vi "Simple Adder Program.vi"() -> ()   [LabVIEW 2018]
uses:
  <vilib>/RTI DDS Toolkit/Types/RTI DDS Advanced Reader Configuration.ctl
  <vilib>/RTI DDS Toolkit/Types/RTI DDS Advanced Writer Configuration.ctl
  <vilib>/RTI DDS Toolkit/VIs/AdvancedCreateWriter_NumI32.vi
  <vilib>/RTI DDS Toolkit/VIs/Write_NumI32.vi
  <vilib>/RTI DDS Toolkit/VIs/AdvancedCreateReader_NumI32.vi
  <vilib>/RTI DDS Toolkit/VIs/Read_NumI32.vi
  <vilib>/RTI DDS Toolkit/Library/LVDDS_library.lvlib
panel:
  out "Int to ROS":i32=7
  in  "error in (no error) 2":errorcluster
  in  "Advanced Writer Configuration":T1={"typeName"="std_msgs::msg::dds_::Int32_", "keyName"="", "domainParticipantQoSProfile"="", "dataWriterQoSProfile"="", "forceArrayMapping?"=FALSE, "forceUnboundedString?"=FALSE}
  in  "stop":bool
  out "Int from ros":i32
  in  "error in (no error)":errorcluster
  in  "Advanced Reader Configuration":T2={"typeName"="std_msgs::msg::dds_::Int32_", "keyName"="", "domainParticipantQoSProfile"="", "dataReaderQoSProfile"="", "forceArrayMapping?"=FALSE, "forceExclusiveReader?"=FALSE, "forceRead? (only ExclusiveReader)"=FALSE, "forceUnboundedString?"=FALSE}
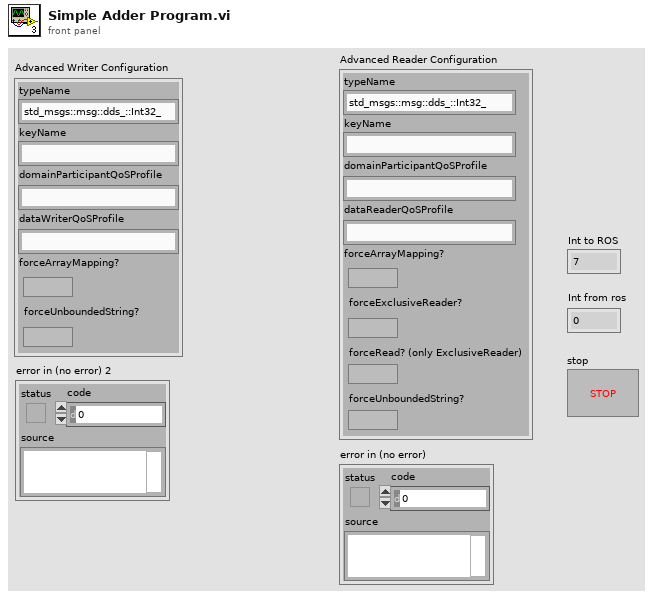
[diagram p1: front panel]
types:
  T1 = typedef "LVDDS_library.lvlib/RTI DDS Advanced Writer Configuration.ctl" = cluster{"typeName":string, "keyName":string, "domainParticipantQoSProfile":string, "dataWriterQoSProfile":string, "forceArrayMapping?":bool, "forceUnboundedString?":bool}
  T2 = typedef "LVDDS_library.lvlib/RTI DDS Advanced Reader Configuration.ctl" = cluster{"typeName":string, "keyName":string, "domainParticipantQoSProfile":string, "dataReaderQoSProfile":string, "forceArrayMapping?":bool, "forceExclusiveReader?":bool, "forceRead? (only ExclusiveReader)":bool, "forceUnboundedString?":bool}
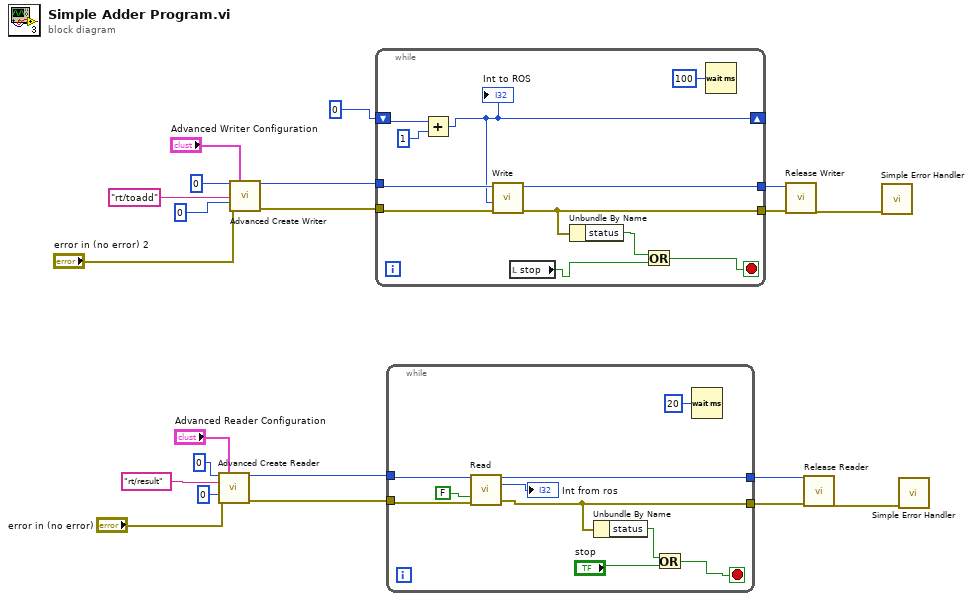
[diagram p0: block diagram]
diagram:
  n1 = call-poly <vilib>:"Advanced Create Reader.vi"("Domain Id"=u32 0 ("Domain id"), "Advanced Reader Configuration"="Advanced Reader Configuration", "Topic Name"="rt/result", "Data Type"=0, "error in (no error)"="error in (no error)") -> ("DDS Object Ref"=w16:u64, "error out"=w15:errorcluster)  [unwired: 9 in]
  n2 = call-poly <vilib>:"Advanced Create Writer.vi"("Domain Id"=u32 0, "Advanced Writer Configuration"="Advanced Writer Configuration", "Topic Name"="rt/toadd", "Data Type"=0, "error in (no error)"="error in (no error) 2") -> ("DDS Object Ref"=w5:u64, "error out"=w4:errorcluster)  [unwired: 9 in]
  n3 = while {
    shift-right: [w27] -> _
    shift-left: 0 -> [w31]
    tunnel: w5 -> [w29]
    tunnel: w4 -> [w28]
    tunnel: [w26] -> w3
    tunnel: [w25] -> w2
    stop <- w23 stop-if-true
    n4 = Add(x=w31, y=1) -> (x+y=w27:i32)
    "Int to ROS" <- w27
    n5 = call-poly <vilib>:"Write.vi"("error in (no error)"=w28, "Data"=w27, "DDS Object Ref in"=w29) -> ("error out"=w25:errorcluster, "DDS Object Ref out"=w26:u64)  [unwired: 7 in]
    n6 = local read "stop"() -> (w22:bool)
    n7 = Unbundle By Name "Unbundle By Name"(w25) -> ("status"=w24:bool)
    n8 = Or(x=w24, y=w22) -> (x .or. y?=w23:bool)
    n9 = Wait (ms)(milliseconds to wait=u32 100) -> ()  [unwired: 1 out]
  }
  n10 = while {
    tunnel: w16 -> [w42]
    tunnel: w15 -> [w41]
    tunnel: [w38] -> w14
    tunnel: [w37] -> w13
    stop <- w34 stop-if-true
    n11 = call-poly <vilib>:"Read.vi"("DDS Object Ref in"=w42, "Only New Samples"=FALSE, "error in (no error)"=w41) -> ("DDS Object Ref out"=w38:u64, "Data"=→"Int from ros":i32, "error out"=w37:errorcluster)  [unwired: 8 in, 2 out]
    n12 = Unbundle By Name(w37) -> ("status"=w36:bool)
    n13 = Or(x=w36, y="stop") -> (x .or. y?=w34:bool)
    n14 = Wait (ms)(milliseconds to wait=u32 20) -> ()  [unwired: 1 out]
  }
  n15 = call <vilib>:"Release Writer.vi"("error in (no error)"=w2, "DDS Object Ref"=w3) -> ("error out"=w1:errorcluster)  [unwired: 9 in]
  n16 = call <vilib>:"Release Reader.vi"("error in (no error)"=w13, "DDS Object Ref"=w14) -> ("error out"=w12:errorcluster)  [unwired: 9 in]
  n17 = call <vilib>:"Simple Error Handler.vi"("error in (no error)"=w1) -> ()  [unwired: 4 in, 5 out]
  n18 = call <vilib>:"Simple Error Handler.vi"("error in (no error)"=w12) -> ()  [unwired: 4 in, 5 out]
